vi "CenterFinderUsingEdges.vi"(0 "Operation":enum16{"Manual", "Automatic"}(ring)=enum."Automatic", 1 "Zone":enum16{"ZoneA", "ZoneB", "ZoneC", "ZoneD"}(ring), 2 "Autofocus":T2={"Enable"=TRUE, "InitialStepSize"=0.05, "Tolerance"=0.02, "Abort"=FALSE} {"Tolerance" format="%#_13g"}, 5 "Component":T4(ring)=enum."BP_CuEdges", 9 "VisibilityInCamera":enum16{"JoyStick", "AllVisible"}(ring)=enum."AllVisible", 11 "error in (no error)":errorcluster, 12 "Position":enum16{"1", "2"}(ring), 13 "SaveImagesLog":bool=TRUE) -> (4 "Output XYZU":string, 6 "Image":T3(plugin-control), 8 "Image 2":T3[](array[plugin-control]) caption="AllImages", 15 "error out":errorcluster)   [LabVIEW 2021]
uses:
  <vilib>/userDefined/High Color/IMAQdx.ctl
  <vilib>/Analysis/coordinate.llb/2D Cartesian Coordinate Rotation (Scalar).vi
  <vilib>/Analysis/baseanly.llb/Mean (DBL).vi
  include/GlobalVariables.vi
  <vilib>/Analysis/NI_AALPro.lvlib
  <vilib>/vision/NI_Vision_Development_Module.lvlib
  <vilib>/Analysis/NI_AALBase.lvlib
  <vilib>/vision/driver/NI_Vision_Acquisition_Software.lvlib
panel:
  out "JoyStickStatus":bool
  in  "Camera":T1="cam1"
  out "Angles":dbl[](array[numeric])
  out "OutputFile":string
  out "spreadsheet string 2":string
  out "spreadsheet string":string
  in  "ModuleName":string="T1"
  out "SyringeY":dbl format="%#_7g"
  out "SyringeX":dbl format="%#_7g"
  in  "CamToSyringeYoffset":dbl=126.651
  in  "CamToSyringeXoffset":dbl=167.702
  out "FileUsedForFiducials":string
  out "UsedCoordinates":string
  out "CameraGcode":string
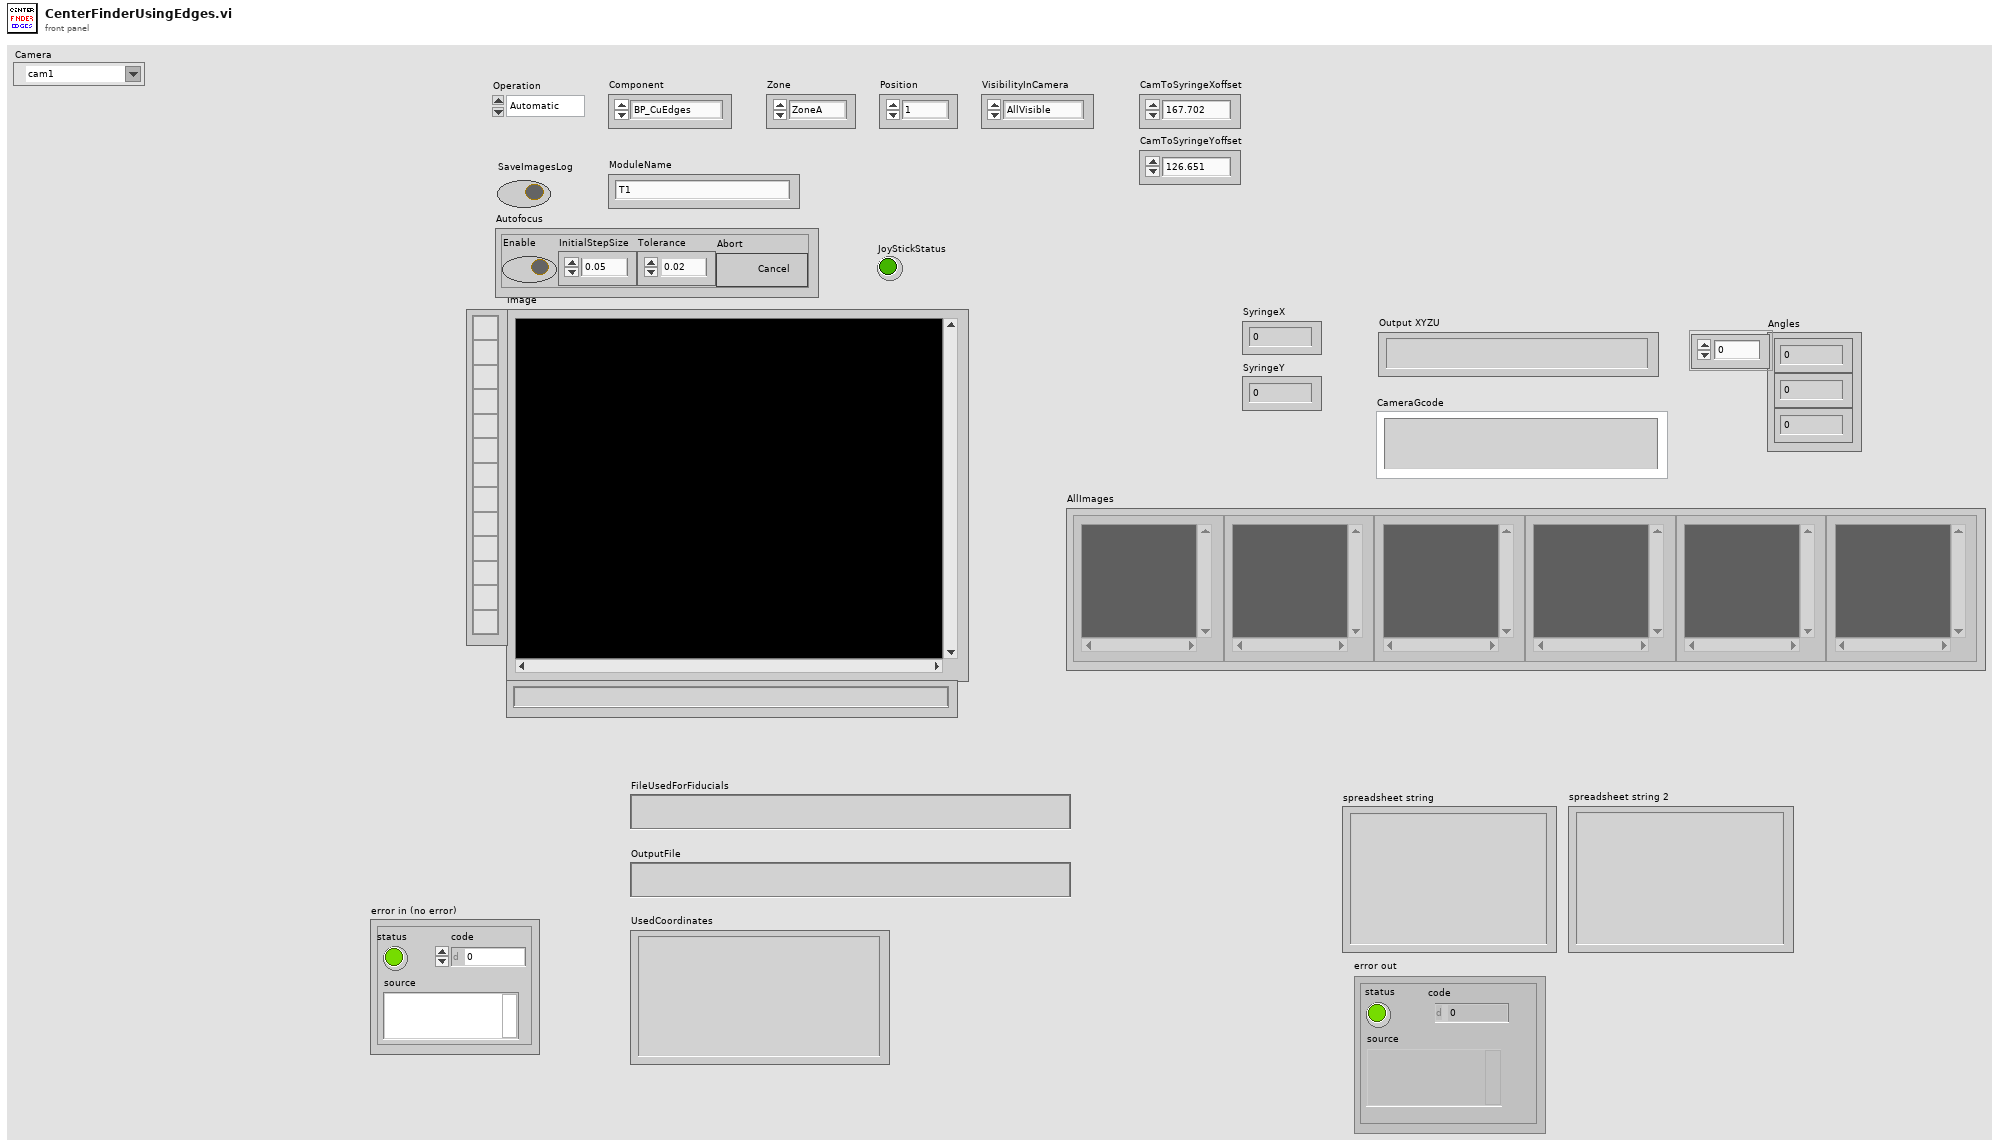
[diagram p1: front panel]
types:
  T1 = typedef "IMAQdx.ctl" = refnum<k21>
  T2 = cluster{"Enable":bool, "InitialStepSize":dbl, "Tolerance":dbl, "Abort":bool}
  T3 = typedef "IMAQ Image.ctl" = refnum<image>
  T4 = enum16{"BP_BackLight", "Si", "SiOnBP", "HB", "HBOnBPSi", "BP_CuEdges", "Other"}
  T5 = cluster{"Number of Matches Requested":i32, "Minimum Match Score":sgl, "Angle Ranges":cluster{"Start Angle":sgl, "End Angle":sgl}[]}
  T6 = typedef "Image Type" = u32
  T7 = typedef "IMAQ Point" = cluster{"X":sgl, "Y":sgl}
  T8 = cluster{"Point 1":cluster{"X":sgl, "Y":sgl}, "Point 2":cluster{"X":sgl, "Y":sgl}}
  T9 = enum16{"Left Button", "Center Button", "Right Button", "Window Close"}
  T10 = enum16{"open", "replace", "create", "open or create", "replace or create", "replace or create with confirmation"}
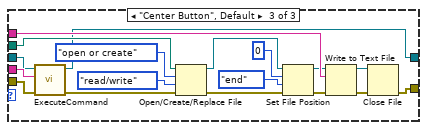
[diagram p4: hidden frame]
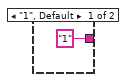
[diagram p5: hidden frame]
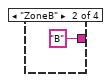
[diagram p6: hidden frame]
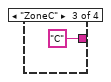
[diagram p7: hidden frame]
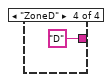
[diagram p8: hidden frame]
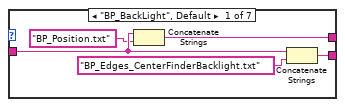
[diagram p9: hidden frame]
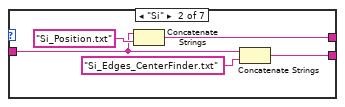
[diagram p10: hidden frame]
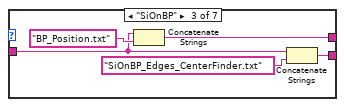
[diagram p11: hidden frame]
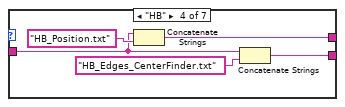
[diagram p12: hidden frame]
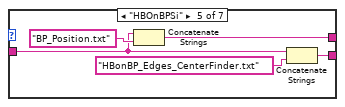
[diagram p13: hidden frame]
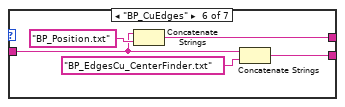
[diagram p14: hidden frame]
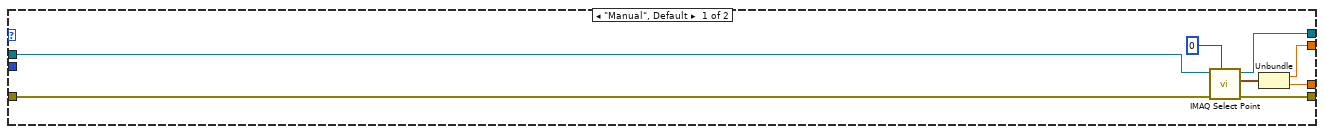
[diagram p15: hidden frame]
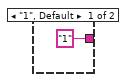
[diagram p17: hidden frame]
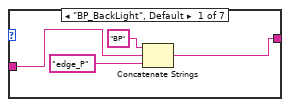
[diagram p18: hidden frame]
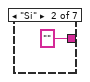
[diagram p19: hidden frame]
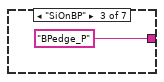
[diagram p20: hidden frame]
diagram:
  w38 = "%f" ("format string")
  w80 = "\t"
  w77 = i16 6 ("width (-)")
  # "Write the XYZU of the baseplate to a text file & move the gantry?"
  # "Prepare to move the gantry to see the center of baseplate in camera."
  # "Find avg X or Y to get the center. \nNote that centrod of equilateral triangle\nconstructed from L1, L2 & L3 is the center of baseplate."
  # "Intersection of L3 & L1"
  # "Intersection of L1 & L2."
  # "Fit line, L1, through pt1 & pt2"
  # "Intersection of L2 & L3"
  # "Fit line, L3, through pt5 & pt6"
  # "Fit line, L2, through pt3 & pt4"
  # "Get (X,Y) for pt3 & pt4"
  # "Get (X,Y) for pt5 & pt6"
  # "Get (X,Y) for pt1 and pt2"
  # "Find the orientation using 1,2,3,4 points (xin[4], yin[4] arrays).\nPoints 5&6 are not used since they may give inifinity in calculation."
  # "AllVisble: Assumes that you know the coordinates of all corners (fiducials) well. No need for any adjustments.\nJoyStick: Use joystick at each point to make good image.\nClickMove: Use \"AdjustCamera\" panel and move the gantry stepwise. Click \"Done\" when you're satisfied with the picture."
  n1 = flat-sequence {
    tunnel: [w120] -> w34
    tunnel: w34 -> [w136]
    tunnel: [w135] -> w33
    tunnel: [w134] -> w31
    tunnel: [w133] -> w28
    tunnel: w33 -> [w198]
    tunnel: [w198] -> w32
    tunnel: w31 -> [w191]
    tunnel: [w186] -> w30
    tunnel: [w197] -> w29
    tunnel: w28 -> [w196]
    tunnel: [w196] -> w27
    tunnel: [w190] -> w12
    tunnel: [w189] -> w11
    tunnel: 6 -> [w225]
    tunnel: "VisibilityInCamera" -> [w218]
    tunnel: w32 -> [w216]
    tunnel: w30 -> [w208]
    tunnel: w29 -> [w215]
    tunnel: w27 -> [w214]
    tunnel: w12 -> [w206]
    tunnel: w11 -> [w207]
    tunnel: [w224] -> w10
    tunnel: [w223] -> w9
    tunnel: [w222] -> w8
    tunnel: [w221] -> w7
    tunnel: [w220] -> w6
    tunnel: [w219] -> w5
    tunnel: [w217] -> w4
    tunnel: [w214] -> w3
    tunnel: [w213] -> w2
    tunnel: [w205] -> w1
    tunnel: [w500] -> w25
    tunnel: [w501] -> w26
    tunnel: [w502] -> w43
    tunnel: [w503] -> w56
    tunnel: [w497] -> w99
    tunnel: [w504] -> w114
    tunnel: [w505] -> w115
    tunnel: [w506] -> w39
    tunnel: [w507] -> w40
    tunnel: w10 -> [w507]
    tunnel: w9 -> [w506]
    tunnel: w8 -> [w505]
    tunnel: w7 -> [w504]
    tunnel: w6 -> [w498]
    tunnel: w5 -> [w503]
    tunnel: w4 -> [w502]
    tunnel: w3 -> [w501]
    tunnel: w2 -> [w500]
    tunnel: w1 -> [w499]
    frame #0 {
      n2 = case shown="\"ZoneA\", Default" "Zone" {
        tunnel: ["A" "B" "C" "D"] -> w124
        frame "ZoneA", Default {
        }
        frame "ZoneB" {
        }
        frame "ZoneC" {
        }
        frame "ZoneD" {
        }
      }
      n3 = case shown="\"2\"" "Position" {
        tunnel: ["1" "2"] -> w125
        frame "1", Default {
        }
        frame "2" {
        }
      }
      n4 = Concatenate Strings(w124, w125, "_" ("string")) -> (w120:string)
      "UsedCoordinates" <- ""
    }
    frame #1 {
      n5 = Concatenate Strings("C:\\Users\\TTUHEP\\Documents\\LabVIEW\\GantryPrograms\\", "Configs\\" ("string"), w136) -> (w143:string)
      n6 = case shown="\"Other\"" "Component" {
        tunnel: w143 -> [w153 w157 w162 w167 w172 w177 w182]
        tunnel: [w154 w159 w164 w169 w174 w179 w184] -> w146
        tunnel: [w151 w156 w161 w166 w171 w176 w181] -> w133
        frame "BP_BackLight", Default {
          n7 = Concatenate Strings(w153, "BP_Position.txt") -> (w151:string)
          n8 = Concatenate Strings(w153, "BP_Edges_CenterFinderBacklight.txt") -> (w154:string)
        }
        frame "Si" {
          n9 = Concatenate Strings(w157, "Si_Position.txt") -> (w156:string)
          n10 = Concatenate Strings(w157, "Si_Edges_CenterFinder.txt") -> (w159:string)
        }
        frame "SiOnBP" {
          n11 = Concatenate Strings(w162, "BP_Position.txt") -> (w161:string)
          n12 = Concatenate Strings(w162, "SiOnBP_Edges_CenterFinder.txt") -> (w164:string)
        }
        frame "HB" {
          n13 = Concatenate Strings(w167, "HB_Position.txt") -> (w166:string)
          n14 = Concatenate Strings(w167, "HB_Edges_CenterFinder.txt") -> (w169:string)
        }
        frame "HBOnBPSi" {
          n15 = Concatenate Strings(w172, "BP_Position.txt") -> (w171:string)
          n16 = Concatenate Strings(w172, "HBonBP_Edges_CenterFinder.txt") -> (w174:string)
        }
        frame "BP_CuEdges" {
          n17 = Concatenate Strings(w177, "BP_Position.txt") -> (w176:string)
          n18 = Concatenate Strings(w177, "BP_EdgesCu_CenterFinder.txt") -> (w179:string)
        }
        frame "Other" {
          n19 = Concatenate Strings(w182, "Other_Position.txt") -> (w181:string)
          n20 = Concatenate Strings(w182, "Other_Edges_CenterFinder.txt") -> (w184:string)
        }
      }
      "FileUsedForFiducials" <- w146
      "OutputFile" <- w133
      n21 = String To Path(string=w146) -> (path=w144:path)
      n22 = Concatenate Strings("This file does not exist:" ("ErrorMessage"), w146) -> (w147:string)
      n23 = call <vilib>:"Check if File or Folder Exists.vi"("error in (no error)"="error in (no error)", "path"=w144) -> ("error out"=w145:errorcluster, "file or folder exists?"=w148:bool, "dup path"=w135:path)  [unwired: 7 in]
      n24 = Not(x=w148) -> (.not. x?=w149:bool)
      n25 = call "AddError.vi"("NoErrorMessage"="InFile OK", "ErrorMessage"=w147, "error in"=w145, "code"=-995, "Error?"=w149) -> ("Error out"=w134:errorcluster)  [unwired: 6 in]
    }
    frame #2 {
      w192 = T6 0 items=["Grayscale (U8)", "Grayscale (I16)", "Grayscale (SGL)", "Complex (CSG)", "RGB (U32)", "HSL (U32)", "RGB (U64)", "Grayscale (U16)"] ("Image Type")
      # "Set the size of the window while selecting the point."
      n26 = call "IMAQ WindSize"("Scrollbars? (N)"=TRUE, "Width & Height"=cluster{"Width":i32, "Height":i32} {"Width"=1333, "Height"=1000}, "Window Number"=0) -> ()  [unwired: 3 in, 3 out]
      n27 = call "IMAQ Create"("Image Name"="name1" ("ImageName"), "Image Type"=w192, "error in (no error)"=w191) -> ("New Image"=w189:T3, "error out"=w194:errorcluster)  [unwired: 2 in]
      n28 = call "Connect.vi"("error in (no error)"=w191) -> ("error out"=w200:errorcluster, "controller"=w201:refnum<k24>)  [unwired: 9 in]
      n29 = call "ExecuteCommand.vi"("error in (no error)"=w200, "Command Code"="G90\nG1 Z0 F100", "controller in"=w201) -> ("error out"=w188:errorcluster, "controller out"=w197:refnum<k24>)  [unwired: 6 in, 1 out]
      n30 = call <vilib>:"IMAQdx Open Camera.vi"("error in"=w194, "Session In"="Camera") -> ("error out"=w187:errorcluster, "Session Out"=w190:T1)  [unwired: 8 in]
      n31 = Merge Errors(w188, w187) -> (w186:errorcluster)
    }
    frame #3 {
      n32 = local read "Autofocus"() -> (w210:T2)
      n33 = local read "Autofocus"() -> (w212:T2)
      n34 = Unbundle By Name(w212) -> ("Enable"=w211:bool)
      n35 = Unbundle By Name(w210) -> ("Abort"=w209:bool)
      n36 = for {
        N: w225 -> [_]
        tunnel: w215 -> [w286]
        tunnel: w216 -> [w269]
        tunnel: [w267] -> w224 mode=indexing
        tunnel: [w266] -> w223 mode=indexing
        tunnel: [w265] -> w222 mode=indexing
        tunnel: [w261] -> w221 mode=indexing
        tunnel: [w260] -> w219
        tunnel: w218 -> [w259]
        tunnel: w209 -> [w258]
        tunnel: w211 -> [w257]
        tunnel: [w253] -> w217
        tunnel: [w248] -> w213 mode=indexing
        shift-right: [w251] -> w220
        shift-left: w208 -> [w235]
        tunnel: w207 -> [w234]
        shift-right: [w228] -> w205
        shift-left: w206 -> [w227]
        i -> [w246]
        w237 = T6 6 items=["Grayscale (U8)", "Grayscale (I16)", "Grayscale (SGL)", "Complex (CSG)", "RGB (U32)", "HSL (U32)", "RGB (U64)", "Grayscale (U16)"] ("Image Type")
        # "Array of XY cluser"
        # "Z array"
        # "Y array"
        # "X array"
        # "Read text file line by line. Each line contains X,Y,Z coordinates for the gantry."
        n37 = call "GetArrayFmTxtFile.vi"("error in"=w235, "LineNo."=w246, "TextFile"=w269) -> ("error out"=w268:errorcluster, "Array"=w293:dbl[])
        n38 = Index Array(array=w293, index=0) -> (element=w288:dbl)
        n39 = Index Array(array=w293, index=1) -> (element=w287:dbl)
        n40 = Index Array(array=w293, index=2) -> (element=w289:dbl)
        n41 = call "Move.vi"("X"=w288, "Absolute"=TRUE, "Y"=w287, "Z"=w289, "SpeedXY (mm/s)"=100.0, "SpeedZ (mm/s)"=100.0, "Move Z first"=FALSE) -> ("Position Gcode"=w285:string)  [unwired: 8 in]
        n42 = call "ExecuteCommand.vi"("error in (no error)"=w268, "Command Code"=w285, "controller in"=w286) -> ("error out"=w233:errorcluster, "controller out"=w284:refnum<k24>)  [unwired: 6 in, 1 out]
        n43 = call <vilib>:"IMAQdx Snap2.vi"("error in"=w233, "Image In"=w234, "Session In"=w227) -> ("error out"=w232:errorcluster, "Image Out"=w230:T3, "Session Out"=w231:T1)  [unwired: 6 in]
        n44 = local write "Image"(w230) -> ()
        n45 = case shown="\"JoyStick\", Default" w259 {
          tunnel: w231 -> [w416 w466]
          tunnel: w284 -> [w432 w478]
          tunnel: w232 -> [w430 w479]
          tunnel: [w412 w467] -> w255
          tunnel: [w420 w473] -> w273
          tunnel: [w421 w471] -> w229
          tunnel: w258 -> [w424 w476]
          tunnel: w257 -> [w418 w477]
          tunnel: "name1" ("ImageName") -> [w417 w465]
          tunnel: w230 -> [w415 w464]
          tunnel: [w411 w463] -> w228
          frame "JoyStick", Default {
            # "Use joystick to go to a position where camera sees good image."
            n46 = while {
              tunnel: [w461] -> w413
              tunnel: w432 -> [w462]
              tunnel: [w459] -> w428
              tunnel: [w462] -> w429
              tunnel: w430 -> [w460]
              tunnel: w416 -> [w458]
              tunnel: w415 -> [w457]
              tunnel: [w456] -> w414
              stop <- w455 continue-if-true
              n47 = call <vilib>:"IMAQdx Snap2.vi"("error in"=w460, "Image In"=w457, "Session In"=w458) -> ("error out"=w459:errorcluster, "Image Out"=w461:T3, "Session Out"=w456:T1)  [unwired: 6 in]
              n48 = local write "Image"(w461) -> ()
              n49 = local read "JoyStickStatus"() -> (w455:bool)
            }
            n50 = call "ExecuteCommand.vi"("error in (no error)"=w430, "Command Code"="JOYSTICK 2D RESET\nJOYSTICK 2D AXISGROUP 1 Y X\nJOYSTICK 2D AXISGROUP 2 Y Z\nJOYSTICK 2D ON", "controller in"=w432) -> ("error out"=w431:errorcluster, "controller out"=w410:refnum<k24>)  [unwired: 6 in, 1 out]
            n51 = call "GetGantryPosition.vi"("error in (no error)"=w428, "Controller In"=w429) -> ("error out"=w409:errorcluster, "controller out"=w423:refnum<k24>, "Position_XYZ"=w419:string)  [unwired: 3 in, 4 out]
            n52 = call <vilib>:"Clear Errors.vi"("error in (no error)"=w431) -> ()  [unwired: 5 in, 2 out]
            n53 = case shown="False" w418 {
              tunnel: w409 -> [w438 w454]
              tunnel: w424 -> [_ w447]
              tunnel: w423 -> [w436 w448]
              tunnel: [w437 w452] -> w422
              tunnel: [w438 w451] -> w421
              tunnel: [w436 w450] -> w420
              tunnel: w419 -> [w437 _]
              tunnel: w417 -> [_ _]
              tunnel: w414 -> [w434 w442]
              tunnel: w413 -> [w435 w441]
              tunnel: [w435 w440] -> w412
              tunnel: [w434 w439] -> w411
              frame False {
              }
              frame True {
                n54 = local read "Autofocus"() -> (w445:T2)
                n55 = Unbundle By Name(w445) -> ("InitialStepSize"=w443:dbl, "Tolerance"=w444:dbl)
                n56 = call "Autofocus.vi"("controller in"=w448, "AbortAutoFocus"=w447, "ImageIn"=w441, "SafeMaxZ"=80.0, "InitialStepSize"=w443, "Tolerance"=w444, "error in (no error)"=w454, "SessionIn"=w442) -> ("controller out"=w453:refnum<k24>, "Image"=w440:T3, "Session Out"=w439:T1, "error out"=w449:errorcluster)  [unwired: 2 in, 2 out]
                n57 = local write "Image"(w440) -> ()
                n58 = call "GetGantryPosition.vi"("error in (no error)"=w449, "Controller In"=w453) -> ("error out"=w451:errorcluster, "controller out"=w450:refnum<k24>, "Position_XYZ"=w452:string)  [unwired: 3 in, 4 out]
              }
            }
            n59 = Not A Number/Path/Refnum?(number/path/refnum=w410) -> (NaN/Path/Refnum?=w408:bool)
            n60 = local write "JoyStickStatus"(w408) -> ()
            n61 = local read "UsedCoordinates"() -> (w426:string)
            n62 = Concatenate Strings(w426, "\r", w422) -> (w427:string)
            n63 = local write "UsedCoordinates"(w427) -> ()
          }
          frame "AllVisible" {
            # "No need to move gantry to take a good pic."
            n64 = case shown="False" w477 {
              tunnel: w476 -> [_ w491]
              tunnel: [w483 w494] -> w472
              tunnel: [w482 w496] -> w474
              tunnel: w479 -> [w483 w495]
              tunnel: w478 -> [w482 w493]
              tunnel: [w481 w490] -> w467
              tunnel: w466 -> [w480 w486]
              tunnel: w465 -> [_ _]
              tunnel: w464 -> [w481 w485]
              tunnel: [w480 w484] -> w463
              frame False {
              }
              frame True {
                n65 = local read "Autofocus"() -> (w489:T2)
                n66 = Unbundle By Name(w489) -> ("InitialStepSize"=w488:dbl, "Tolerance"=w487:dbl)
                n67 = call "Autofocus.vi"("controller in"=w493, "AbortAutoFocus"=w491, "ImageIn"=w485, "SafeMaxZ"=80.0, "InitialStepSize"=w488, "Tolerance"=w487, "error in (no error)"=w495, "SessionIn"=w486) -> ("controller out"=w496:refnum<k24>, "Image"=w490:T3, "Session Out"=w484:T1, "error out"=w494:errorcluster)  [unwired: 2 in, 2 out]
                n68 = local write "Image"(w490) -> ()
              }
            }
            n69 = local read "UsedCoordinates"() -> (w469:string)
            n70 = call "GetGantryPosition.vi"("error in (no error)"=w472, "Controller In"=w474) -> ("error out"=w471:errorcluster, "controller out"=w473:refnum<k24>, "Position_XYZ"=w470:string)  [unwired: 3 in, 4 out]
            n71 = Concatenate Strings(w469, "\r", w470) -> (w468:string)
            n72 = local write "UsedCoordinates"(w468) -> ()
          }
        }
        n73 = case shown="\"Automatic\"" "Operation" {
          tunnel: [w302 w312] -> w281
          tunnel: [w301 w311] -> w280
          tunnel: [w300 w320] -> w279
          tunnel: w229 -> [w299 w337]
          tunnel: w255 -> [w298 w344]
          tunnel: w246 -> [_ w341]
          tunnel: [w297 w318] -> w247
          frame "Manual", Default {
            n74 = call "IMAQ Select Point"("Window Number (0...15)"=0, "error in (no error)"=w299, "Image In"=w298) -> ("error out"=w300:errorcluster, "Point"=w303:T7, "Image Out (duplicate)"=w297:T3)  [unwired: 5 in, 1 out]
            n75 = Unbundle(w303) -> ("X"=w302:sgl, "Y"=w301:sgl)
          }
          frame "Automatic" {
            w316 = sgl 50.0 ("y")
            w335 = ""
            n76 = local read "Position"() -> (w323:enum16{"1", "2"})
            n77 = case shown="\"2\"" w323 {
              tunnel: ["1" "2"] -> w322
              frame "1", Default {
              }
              frame "2" {
              }
            }
            n78 = local read "Component"() -> (w340:T4)
            n79 = case shown="\"BP_CuEdges\"" w340 {
              tunnel: [w361 "" "BPedge_P" "HBedge_P" "HBedge_P" w367 "BPedge_P"] -> w339
              tunnel: w322 -> [w362 _ _ _ _ w368 _]
              frame "BP_BackLight", Default {
                n80 = Concatenate Strings("BP", w362, "edge_P") -> (w361:string)
              }
              frame "Si" {
              }
              frame "SiOnBP" {
              }
              frame "HB" {
              }
              frame "HBOnBPSi" {
              }
              frame "BP_CuEdges" {
                n81 = Concatenate Strings("BP", w368, "CuEdge_P") -> (w367:string)
              }
              frame "Other" {
              }
            }
            n82 = Number To Decimal String(number=w341) -> (decimal integer string=w338:string)  [unwired: 1 in]
            n83 = Concatenate Strings(w339, w338) -> (w330:string)
            n84 = Concatenate Strings("Could not parse/find this template file for pattern recognition:" ("ErrorMessage"), w330) -> (w329:string)
            n85 = call "JSONfileReader.vi"("error in"=w337, "Variant"=w335, "ItemName"=w330, "FileIn"=path "C:/Users/TTUHEP/Documents/LabVIEW/GantryPrograms/Configs/PatternRecognTemplateMaps.json" ("PatterRecognTemplateMap")) -> ("error out"=w326:errorcluster, "Data"=w336:variant, "Found"=w333:bool)
            n86 = Not(x=w333) -> (.not. x?=w332:bool)
            n87 = Variant To Data(error in=w326, type=w335, Variant=w336) -> (data=w334:string, error out=w325:errorcluster)
            n88 = call "AddError.vi"("NoErrorMessage"="Template file name found from json.", "ErrorMessage"=w329, "error in"=w325, "code"=-902, "Error?"=w332) -> ("Error out"=w324:errorcluster)  [unwired: 6 in]
            n89 = call "PatternRecognition.vi"("error in (no error)"=w324, "MatchParameters"=T5 {"Number of Matches Requested"=1, "Minimum Match Score"=800.0, "Angle Ranges"=[{"Start Angle"=0.0, "End Angle"=0.0}]}, "ImageIn"=w344, "TemplateFileName"=w334) -> ("error out"=w307:errorcluster, "Position"=w343:cluster{"x":sgl, "y":sgl}, "ImageFoundPattern"=w319:T3, "Number of Matches"=w321:i32)  [unwired: 2 in, 1 out]
            n90 = Equal To 0?(x=w321) -> (x = 0?=w317:bool)
            n91 = Unbundle(w343) -> ("x"=w310:sgl, "y"=w309:sgl)
            n92 = call <vilib>:"Clear Errors.vi"("error in (no error)"=w307, "specific error code to clear (0: all)"=-903) -> ("error out"=w306:errorcluster)  [unwired: 4 in, 1 out]
            n93 = Less?(x=w310, y=w316) -> (x < y?=w315:bool)
            n94 = Less?(x=w309, y=w316) -> (x < y?=w314:bool)
            n95 = Compound Arithmetic op=OR(w317, w315, w314) -> (w313:bool)
            n96 = case shown="True" w313 {
              tunnel: w306 -> [w348 w355]
              tunnel: [w348 w354] -> w320
              tunnel: w319 -> [w347 w353]
              tunnel: [w347 w352] -> w318
              tunnel: [w346 w350] -> w312
              tunnel: [w345 w349] -> w311
              tunnel: w310 -> [w346 _]
              tunnel: w309 -> [w345 _]
              frame False {
              }
              frame True {
                n97 = call "IMAQ Select Point"("Window Number (0...15)"=0, "error in (no error)"=w355, "Image In"=w353) -> ("error out"=w354:errorcluster, "Point"=w351:T7, "Image Out (duplicate)"=w352:T3)  [unwired: 5 in, 1 out]
                n98 = Unbundle(w351) -> ("X"=w350:sgl, "Y"=w349:sgl)
              }
            }
          }
        }
        n99 = Number To Decimal String(number=w246) -> (decimal integer string=w245:string)  [unwired: 1 in]
        n100 = Concatenate Strings("imgTemp" ("string"), w245) -> (w242:string)
        n101 = call "GetPixelToGantryRelPosition.vi"("error in (no error)"=w279, "PixelY"=w280, "PixelX"=w281) -> ("error out"=w240:errorcluster, "YmmRelGH"=w277:dbl, "XmmRelGH"=w278:dbl)
        n102 = call "IMAQ Create"("Image Name"=w242, "Image Type"=w237, "error in (no error)"=w240) -> ("New Image"=w241:T3, "error out"=w239:errorcluster)  [unwired: 2 in]
        n103 = call "IMAQ Copy"("error in (no error)"=w239, "Image Dst"=w241, "Image Src"=w247) -> ("error out"=w238:errorcluster, "Image Dst Out"=w243:T3)  [unwired: 3 in]
        n104 = Build Array(w243) -> (w248:T3[])
        n105 = flat-sequence {
          tunnel: w238 -> [w399]
          tunnel: [w399] -> w283
          tunnel: w273 -> [w398]
          tunnel: [w398] -> w282
          tunnel: [w407] -> w252
          tunnel: [w406] -> w276
          tunnel: [w405] -> w275
          tunnel: [w404] -> w260
          tunnel: [w403] -> w274
          tunnel: w283 -> [w402]
          tunnel: w282 -> [w401]
          frame #0 {
            n106 = Wait (ms)(milliseconds to wait=u32 1000) -> ()  [unwired: 1 out]
          }
          frame #1 {
            n107 = call "GetGantryPosition.vi"("error in (no error)"=w402, "Controller In"=w401) -> ("error out"=w407:errorcluster, "Position Y"=w406:dbl, "Position X"=w405:dbl, "controller out"=w404:refnum<k24>, "Position Z"=w403:dbl)  [unwired: 3 in, 2 out]
          }
        }
        n108 = Add(x=w278, y=w275) -> (x+y=w272:dbl)
        n109 = Add(x=w277, y=w276) -> (x+y=w271:dbl)
        n110 = case shown="True" "SaveImagesLog" {
          tunnel: w247 -> [w372 w390]
          tunnel: w246 -> [_ w388]
          tunnel: ["" w380] -> w253
          tunnel: w252 -> [w373 w379]
          tunnel: [w373 w378] -> w251
          tunnel: [w372 w377] -> w236
          frame False {
          }
          frame True {
            w382 = "C:\\Users\\TTUHEP\\Documents\\LabVIEW\\GantryPrograms\\LogFiles\\CalibrationData\\"
            n111 = local read "Component"() -> (w376:T4)
            n112 = case shown="\"BP_CuEdges\"" w376 {
              tunnel: ["BP_edge" "Si" "SiOnBP" "HB" "HBOnSi" "BP_CuEdge" "Other"] -> w375
              frame "BP_BackLight", Default {
              }
              frame "Si" {
              }
              frame "SiOnBP" {
              }
              frame "HB" {
              }
              frame "HBOnBPSi" {
              }
              frame "BP_CuEdges" {
              }
              frame "Other" {
              }
            }
            n113 = Number To Decimal String(number=w388) -> (decimal integer string=w386:string)  [unwired: 1 in]
            n114 = Concatenate Strings(w382, "ModuleName") -> (w380:string)
            n115 = Concatenate Strings(w382, "ModuleName", w375, "Image" ("string"), w386, ".png" ("string")) -> (w384:string)
            n116 = String To Path(string=w384) -> (path=w383:path)
            n117 = call-poly "IMAQ Write File 2"("error in (no error)"=w379, "Image Quality"=u32 1000, "File Path"=w383, "Image"=w390) -> ("error out"=w378:errorcluster, "Image Out (duplicate)"=w377:T3)  [unwired: 6 in]
          }
        }
        "Image" <- w236
        n118 = call-poly <vilib>:"2D Cartesian Coordinate Rotation.vi"("theta"=0.0, "y"=w271, "x"=w272) -> ("y out"=w263:dbl, "x out"=w264:dbl)  [unwired: 6 in, 1 out]
        n119 = Bundle("x out"=w264, "y out"=w263) -> (w262:cluster{"x out":dbl, "y out":dbl})  [unwired: 1 in]
        n120 = global write "GlobalVariables.vi" "Image"(w236) -> ()
        n121 = Build Array(w262) -> (w261:cluster{"x out":dbl, "y out":dbl}[])
        n122 = Build Array(w263) -> (w266:dbl[])
        n123 = Build Array(w264) -> (w267:dbl[])
        n124 = Build Array(w274) -> (w265:dbl[])
        "JoyStickStatus" <- TRUE ("NaN/Path/Refnum?")
      }
    }
    frame #4 {
      n125 = call <vilib>:"IMAQdx Close Camera.vi"("error in"=w498, "Session In"=w499) -> ("error out"=w497:errorcluster)  [unwired: 9 in]
    }
  }
  n126 = Array To Spreadsheet String(array=w40, 3:w38) -> (spreadsheet string=→"spreadsheet string":string)  [unwired: 1 in]
  n127 = Array To Spreadsheet String(array=w39, 3:w38) -> (spreadsheet string=→"spreadsheet string 2":string)  [unwired: 1 in]
  n128 = String To Path(string=w26) -> (path=w35:path)
  n129 = Index Array(array=w25, index (col)=0 ("disabled index (col)")) -> (element=→"Image 2":T3[])  [unwired: 1 in]
  n130 = Index Array "Y"(array=w39, index (col)=0 ("disabled index (col)")) -> (element=w83:dbl[])  [unwired: 1 in]
  n131 = Index Array "X"(array=w40, index (col)=0 ("disabled index (col)")) -> (element=w84:dbl[])  [unwired: 1 in]
  n132 = Index Array "Z"(array=w115, index (col)=0 ("disabled index (col)")) -> (element=w85:dbl[])  [unwired: 1 in]
  n133 = Index Array "Points"(array=w114, index (col)=0 ("disabled index (col)")) -> (element=w103:cluster{"x out":dbl, "y out":dbl}[])  [unwired: 1 in]
  n134 = formula code="float64 m1 = 0.0, m2 = 0.0, m3 = 0.0;\nfloat64 orientn = 0.0;\nfloat64 angls[3];\nangls[0] = 0.0; angls[1] = 0.0; angls[2] = 0.0;\n\nm1 = (yin[0] - yin[1]) / (xin[0] - xin[1]);\nm2 = (yin[3] - yin[2]) / (xin[3] - xin[2]);\nm3 = (yin[5] - yin[4]) / (xin[5] - xin[4]);\n\nangls[0] = (atan(m1)*180.0/3.14159) - (30.0);\nangls[1] = (atan(m2)*180.0/3.14159) - (-30.0);\nangls[2] = -(atan(1.0/m3)*180.0/3.14159);\n\norientn = (angls[0] + angls[1])/2.0;"("xin"=w84, "yin"=w83) -> ("orientn"=w57:dbl, "angls"=→"Angles":dbl[])
  n135 = Array Subset(array=w103, index=2, length=2) -> (w107:cluster{"x out":dbl, "y out":dbl}[])
  n136 = Array Subset(array=w103, index=0, length=2) -> (w110:cluster{"x out":dbl, "y out":dbl}[])
  n137 = call "IMAQ Fit Line"("error in (no error)"=w99, "Points"=w110) -> ("error out"=w21:errorcluster, "Line Segment"=w100:T8)  [unwired: 4 in, 4 out]
  n138 = call "IMAQ Fit Line"("error in (no error)"=w21, "Points"=w107) -> ("error out"=w20:errorcluster, "Line Segment"=w102:T8)  [unwired: 4 in, 4 out]
  n139 = Array Subset(array=w103, index=4, length=2) -> (w104:cluster{"x out":dbl, "y out":dbl}[])
  n140 = call "IMAQ Fit Line"("error in (no error)"=w20, "Points"=w104) -> ("error out"=w19:errorcluster, "Line Segment"=w101:T8)  [unwired: 4 in, 4 out]
  n141 = call "IMAQ Lines Intersection"("error in (no error)"=w19, "Line 2"=w102, "Line 1"=w100) -> ("error out"=w18:errorcluster, "Intersection Point"=w88:cluster{"X":sgl, "Y":sgl})  [unwired: 6 in, 1 out]
  n142 = Unbundle(w88) -> ("X"=w98:sgl, "Y"=w91:sgl)
  n143 = call "IMAQ Lines Intersection"("error in (no error)"=w18, "Line 2"=w100, "Line 1"=w101) -> ("error out"=w17:errorcluster, "Intersection Point"=w87:cluster{"X":sgl, "Y":sgl})  [unwired: 6 in, 1 out]
  n144 = Unbundle(w87) -> ("X"=w97:sgl, "Y"=w90:sgl)
  n145 = call "IMAQ Lines Intersection"("error in (no error)"=w17, "Line 2"=w101, "Line 1"=w102) -> ("error out"=w16:errorcluster, "Intersection Point"=w86:cluster{"X":sgl, "Y":sgl})  [unwired: 6 in, 1 out]
  n146 = Unbundle(w86) -> ("X"=w96:sgl, "Y"=w89:sgl)
  n147 = call-poly <vilib>:"Mean.vi"("X"=w85) -> ("mean"=w58:dbl)  [unwired: 1 out]
  n148 = Compound Arithmetic op=ADD(w98, w97, w96) -> (w95:sgl)
  n149 = Compound Arithmetic op=ADD(w91, w90, w89) -> (w93:sgl)
  n150 = Divide(x=w93, y=sgl 3.0) -> (x/y=w59:sgl)
  n151 = Divide(x=w95, y=sgl 3.0) -> (x/y=w60:sgl)
  n152 = Number To Fractional String(number=w60, precision (6)=w77) -> (F-format string=w82:string)  [unwired: 2 in]
  n153 = Number To Fractional String(number=w59, precision (6)=w77) -> (F-format string=w81:string)  [unwired: 2 in]
  n154 = Number To Fractional String(number=w58, precision (6)=w77) -> (F-format string=w76:string)  [unwired: 2 in]
  n155 = call "CameraXYusingGantryHeadXY.vi"("GantryY"=w59, "GantryX"=w60) -> ("CamY"=w49:dbl, "CamX"=w51:dbl)
  n156 = Number To Fractional String(number=w57, precision (6)=i16 4 ("width (-)")) -> (F-format string=w78:string)  [unwired: 2 in]
  n157 = call "Move.vi"("X"=w51, "Absolute"=TRUE, "Y"=w49, "Z"=w58, "SpeedXY (mm/s)"=100.0, "SpeedZ (mm/s)"=50.0, "Move Z first"=TRUE) -> ("Position Gcode"=w63:string)  [unwired: 8 in]
  "CameraGcode" <- w63
  n158 = Add(x="CamToSyringeYoffset", y=w49) -> (x+y=→"SyringeY":dbl)
  n159 = Concatenate Strings(w82, w80, w81, w80, w76, w80, w78, "\r") -> (w74:string)
  "Output XYZU" <- w74
  n160 = Add(x="CamToSyringeXoffset", y=w51) -> (x+y=→"SyringeX":dbl)
  n161 = Concatenate Strings("Overwrite/Append ", w74, " to file ", w26, " ?" ("string")) -> (w71:string)
  n162 = call <vilib>:"Three Button Dialog.vi"("Right Button Text (\"Cancel\")"="Do nothing" ("Right Button Text (\"Cancel\")"), "Center Button Text (\"No\")"="Append" ("Center Button Text (\"No\")"), "Left Button Text (\"Yes\")"="Overwrite" ("Left Button Text (\"Yes\")"), "message"=w71) -> ("Which Button?"=w70:T9)  [unwired: 7 in]
  n163 = case shown="\"Left Button\"" w70 {
    tunnel: w74 -> [w515 _ w537]
    tunnel: w35 -> [w514 _ w536]
    tunnel: w16 -> [w513 w523 w535]
    tunnel: w63 -> [w512 _ w534]
    tunnel: w56 -> [w511 w522 w533]
    tunnel: [w508 w523 w524] -> w45
    tunnel: [w510 w522 w532] -> w62
    frame "Left Button" {
      n164 = call "ExecuteCommand.vi"("error in (no error)"=w513, "Command Code"=w512, "controller in"=w511) -> ("error out"=w509:errorcluster, "controller out"=w510:refnum<k24>)  [unwired: 6 in, 1 out]
      n165 = Open/Create/Replace File(file path (use dialog)=w514, error in=w509, operation (0:open)=T10."replace or create", access (0:read/write)=enum16{"read/write", "read-only", "write-only"}."read/write") -> (refnum out=w521:refnum<file>, error out=w518:errorcluster)  [unwired: 2 in, 1 out]
      n166 = Write to Text File(file (use dialog)=w521, text=w515, error in=w518) -> (refnum out=w516:refnum<file>, error out=w517:errorcluster)  [unwired: 1 in, 1 out]
      n167 = Close File(refnum=w516, error in=w517) -> (error out=w508:errorcluster)  [unwired: 1 out]
    }
    frame "Right Button" {
    }
    frame "Center Button", Default {
      n168 = call "ExecuteCommand.vi"("error in (no error)"=w535, "Command Code"=w534, "controller in"=w533) -> ("error out"=w525:errorcluster, "controller out"=w532:refnum<k24>)  [unwired: 6 in, 1 out]
      n169 = Open/Create/Replace File(file path (use dialog)=w536, error in=w525, operation (0:open)=T10."open or create", access (0:read/write)=enum16{"read/write", "read-only", "write-only"}."read/write") -> (refnum out=w529:refnum<file>, error out=w527:errorcluster)  [unwired: 2 in, 1 out]
      n170 = Set File Position(offset (in bytes) (0)=i64 0, refnum=w529, from (0:start)=enum16{"start", "end", "current"}."end", error in=w527) -> (refnum out=w528:refnum<file>, error out=w526:errorcluster)
      n171 = Write to Text File(file (use dialog)=w528, text=w537, error in=w526) -> (refnum out=w538:refnum<file>, error out=w539:errorcluster)  [unwired: 1 in, 1 out]
      n172 = Close File(refnum=w538, error in=w539) -> (error out=w524:errorcluster)  [unwired: 1 out]
    }
  }
  n173 = call "CaptureImage.vi"("Camera"=T1 "cam1", "ImageName"="CurrImage", "Draw50MicroCircleAtCenter"=TRUE, "error in (no error)"=w45) -> ("Image"=w22:T3, "error out"=w44:errorcluster)  [unwired: 3 in]
  n174 = local write "Image"(w22) -> ()
  n175 = global write "GlobalVariables.vi" "Image"(w22) -> ()
  n176 = call "Disconnect.vi"("error in (no error)"=w44, "controller"=w62) -> ("error out"=w41:errorcluster)  [unwired: 9 in]
  n177 = local read "SaveImagesLog"() -> (w46:bool)
  n178 = case shown="True" w46 {
    tunnel: w41 -> [w542 w557]
    tunnel: w43 -> [_ w550]
    tunnel: w22 -> [_ w545]
    tunnel: [w542 w543] -> w42
    frame False {
    }
    frame True {
      n179 = Concatenate Strings(w550, "UsedXYZ.txt") -> (w555:string)
      n180 = local read "UsedCoordinates"() -> (w552:string)
      n181 = Concatenate Strings(w550, "CenterImage.png") -> (w548:string)
      n182 = String To Path(string=w555) -> (path=w554:path)
      n183 = String To Path(string=w548) -> (path=w546:path)
      n184 = Open/Create/Replace File(file path (use dialog)=w554, error in=w557, operation (0:open)=T10."open or create", access (0:read/write)=enum16{"read/write", "read-only", "write-only"}."read/write") -> (refnum out=w553:refnum<file>, error out=w561:errorcluster)  [unwired: 2 in, 1 out]
      n185 = Write to Text File(file (use dialog)=w553, text=w552, error in=w561) -> (refnum out=w551:refnum<file>, error out=w560:errorcluster)  [unwired: 1 in, 1 out]
      n186 = Close File(refnum=w551, error in=w560) -> (error out=w544:errorcluster)  [unwired: 1 out]
      n187 = call-poly "IMAQ Write File 2"("error in (no error)"=w544, "Image Quality"=u32 1000, "File Path"=w546, "Image"=w545) -> ("error out"=w543:errorcluster)  [unwired: 6 in, 1 out]
    }
  }
  "error out" <- w42
